vi "禹山溶解氧校准.vi"() -> ()   [LabVIEW 2016, in "斯坦道多参数.lvlib"]
uses:
  <vilib>/Utility/miscctls.llb/LVPointTypeDef.ctl
  <vilib>/Analysis/NI_AALBase.lvlib
  <vilib>/Analysis/NI_AALPro.lvlib
  <vilib>/Utility/config.llb/NI_LVConfig.lvlib
panel:
  out "通讯状态":string
  in  "盐度自动获取":bool
  in  "大气压补偿":dbl format="%#.2f"
  in  "盐度补偿":dbl format="%#.2f"
  out "DO %":dbl caption="饱和度值" format="%#.2f"
  out "第二点校准值":dbl
  out "第一点校准值":dbl
  out "最小值":sgl format="%.2g"
  out "最大值":sgl format="%.2g"
  in  "校准停止":bool
  in  "校准模式":enum16{"两点校准", "单点校准"}(ring)
  in  "标液2":dbl
  in  "标液1":dbl
  out "波形图表":sgl(graph) caption="历史曲线"
  out "温度测量值":dbl caption="温度" format="%#.2f"
  out "变异系数":dbl format="%.6g"
  out "standard deviation":dbl caption="标准差" format="%0.2f"
  out "mean":dbl caption="均值" format="%0.2f"
  out "提示":string
  in  "校准启动":bool
  out "DO mg/L":dbl caption="测试值" format="%#.2f"
  out "电极斜率":dbl format="%#.6f"
  out "电极零点":dbl format="%#.6f"
  # "溶解氧电极设定"
  # "℃"
  # "%"
  # "mg/L"
  # "kPa"
  # "请选择校准模式:"
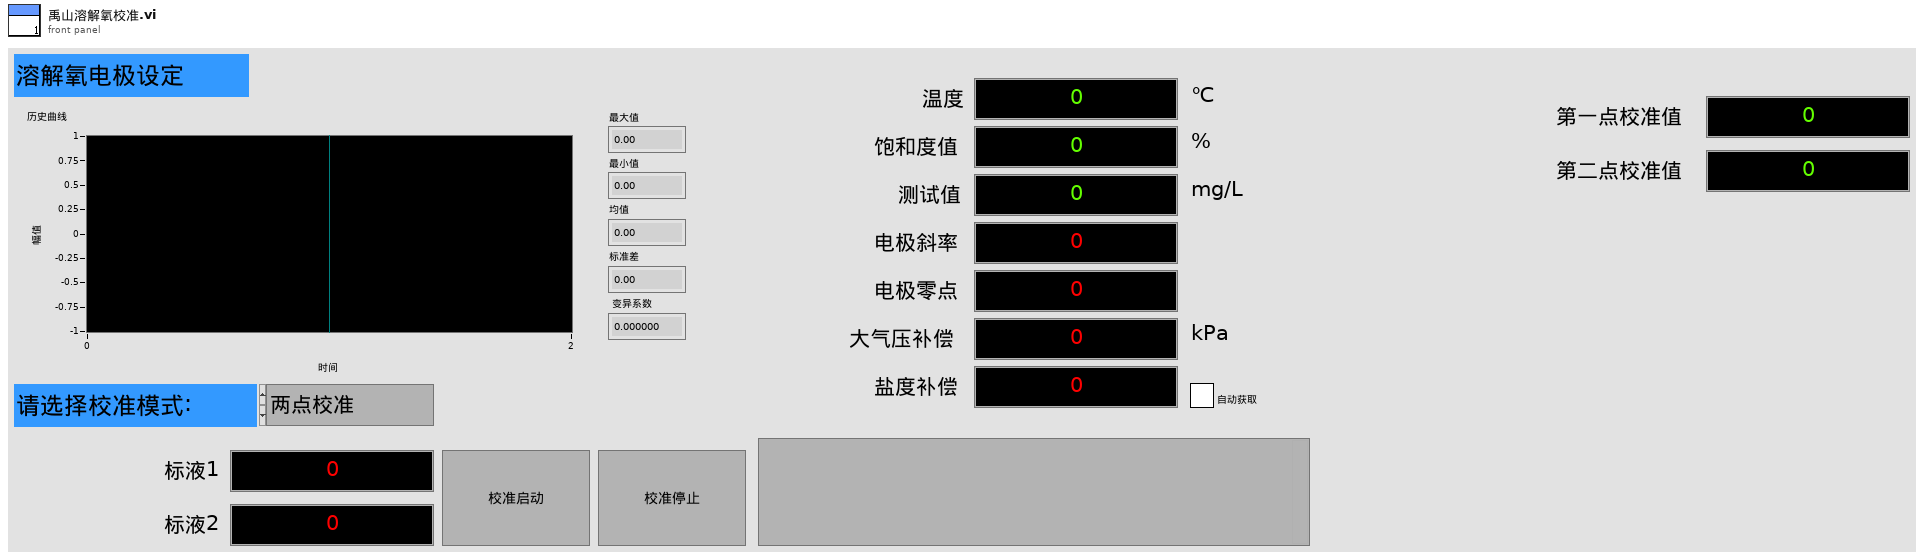
[diagram p1: front panel]
types:
  T1 = typedef "斯坦道多参数.lvlib/校准步骤.ctl" = enum16{"待机", "放置第一点标液", "第一点校准启动", "第一点校准写入", "第一点校准失败", "放置第二点标液", "第二点校准启动", "第二点校准写入", "第二点校准失败", "放置第三点标液", "第三点校准启动", "第三点校准写入", "第三点校准失败", "校准结果写入", "校准结束"}
  T2 = typedef "LVPointTypeDef.ctl" = cluster{"Horizontal":i16, "Vertical":i16}
  T3 = typedef "NI_LVConfig.lvlib/Config Data RefNum.ctl" = refnum<k1>
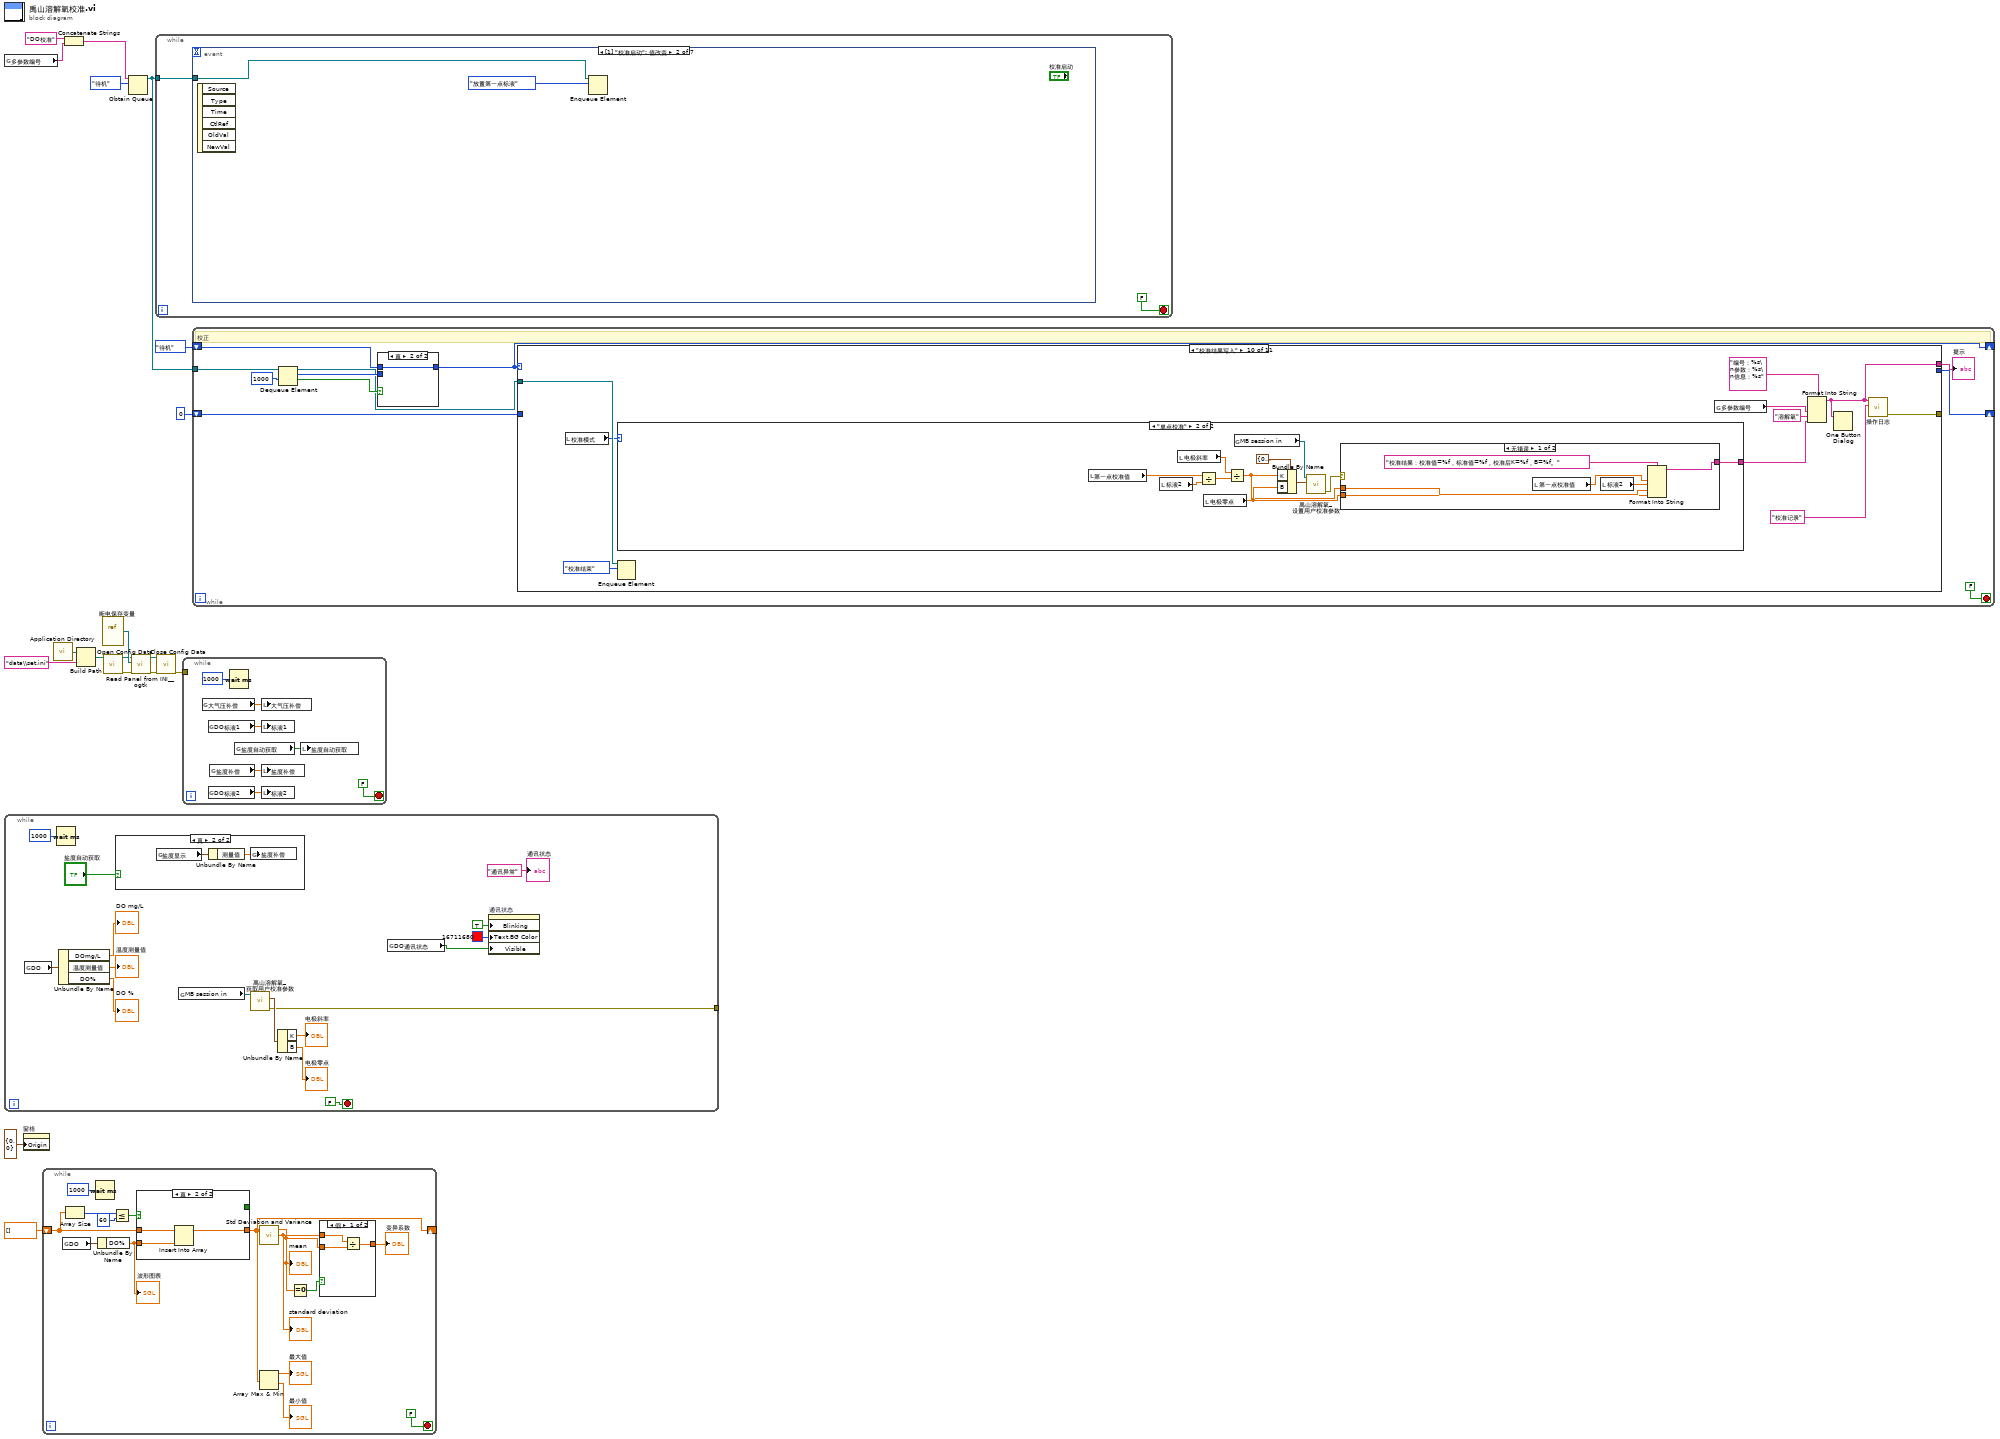
[diagram p0: block diagram]
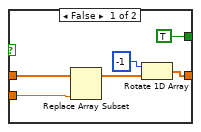
[diagram p3: hidden frame]
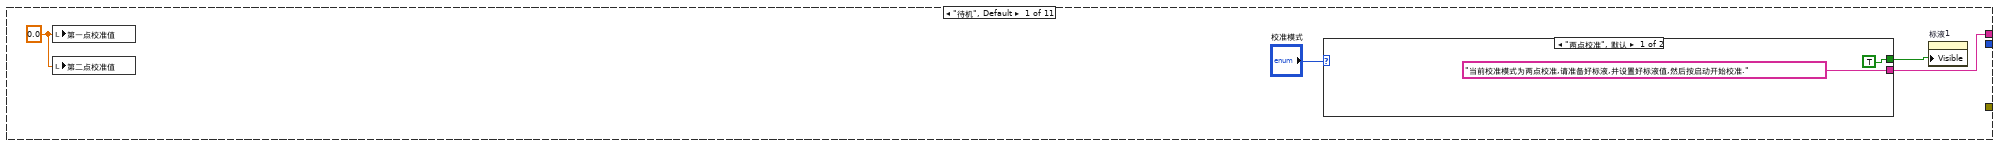
[diagram p5: hidden frame]
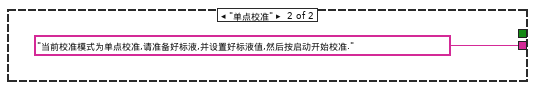
[diagram p6: hidden frame]
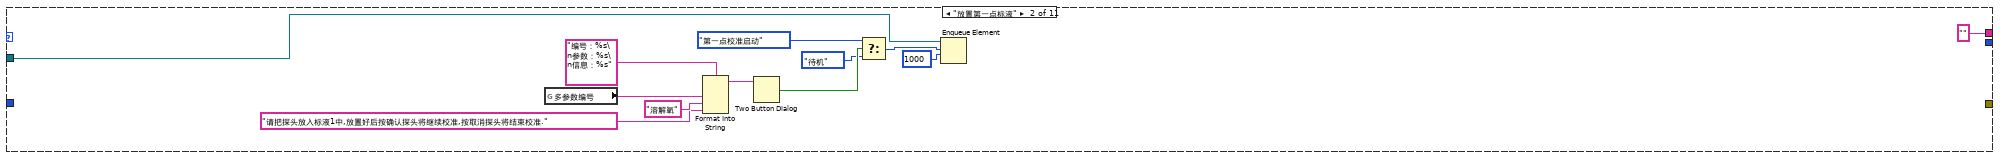
[diagram p7: hidden frame]
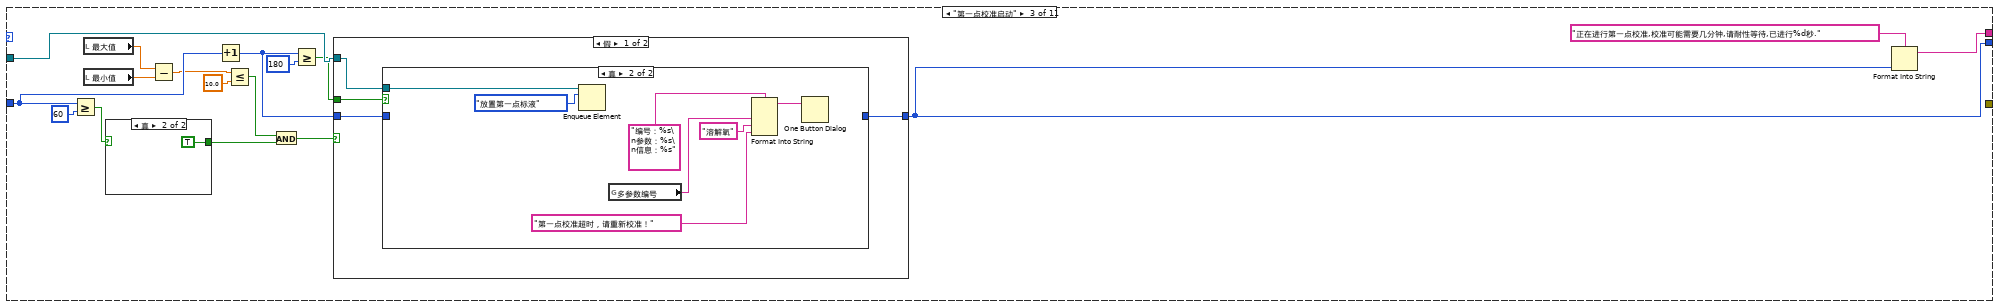
[diagram p8: hidden frame]
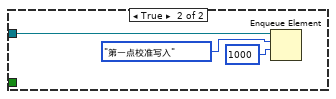
[diagram p10: hidden frame]
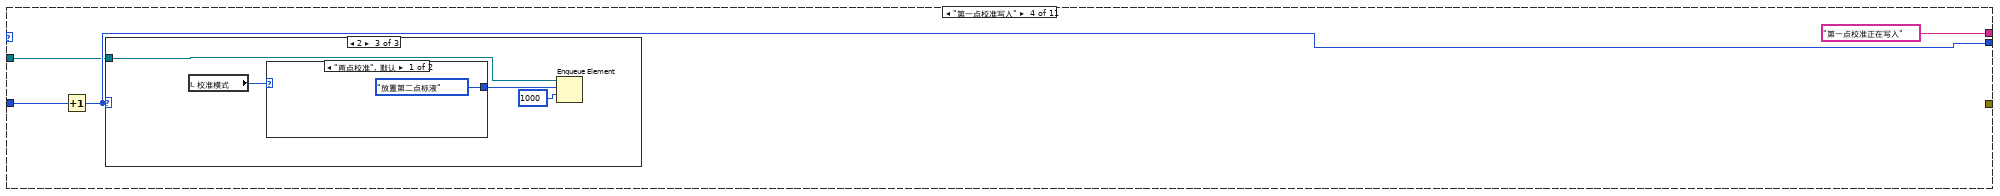
[diagram p12: hidden frame]
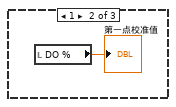
[diagram p14: hidden frame]
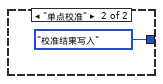
[diagram p15: hidden frame]
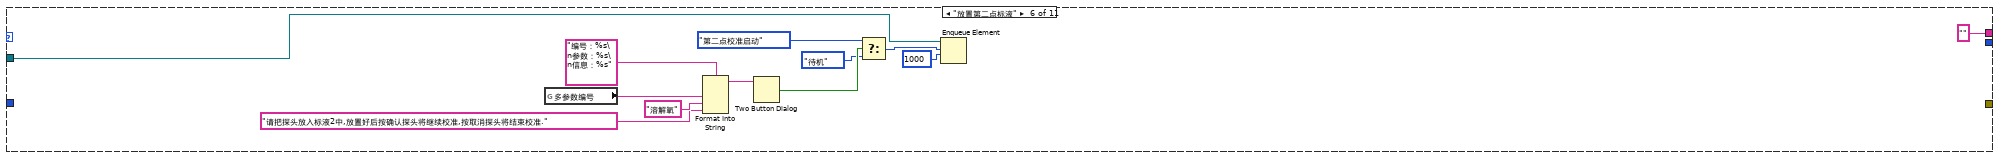
[diagram p17: hidden frame]
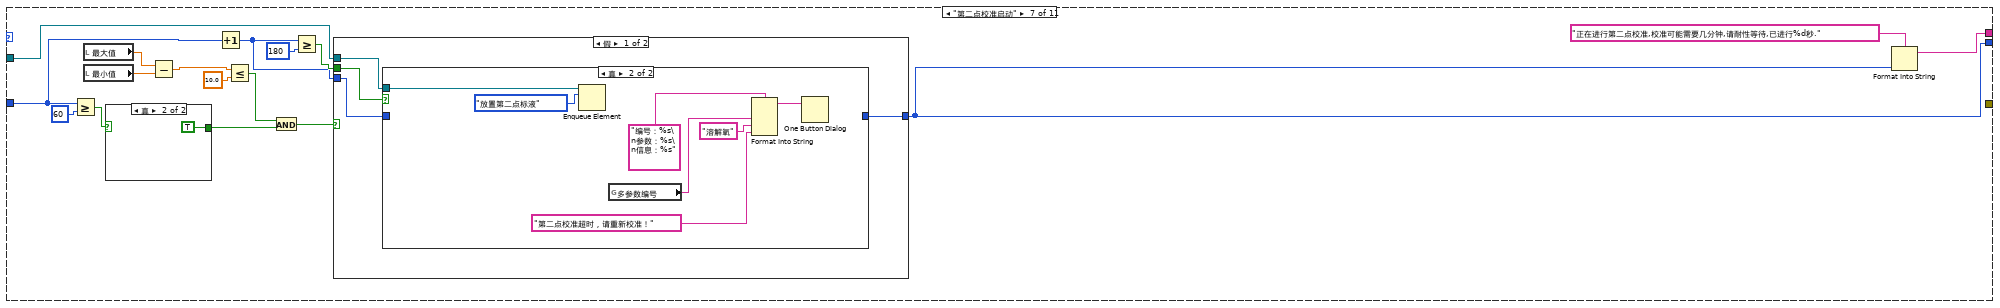
[diagram p18: hidden frame]
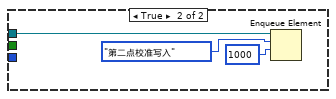
[diagram p20: hidden frame]
diagram:
  n1 = global read "多参数全局变量.vi" "多参数编号"() -> (w1:string)
  n2 = while {
    tunnel: [w29] -> _
    stop <- FALSE stop-if-true
    n3 = global read "禹山过程全局变量.vi" "DO"() -> (w26:cluster{"温度测量值":sgl, "DO%":sgl, "DOmg/L":sgl})
    n4 = Wait (ms)(milliseconds to wait=u32 1000 ("等待时间（毫秒）")) -> ()  [unwired: 1 out]
    n5 = Unbundle By Name(w26) -> ("DOmg/L"=→"DO mg/L":sgl, "温度测量值"=→"温度测量值":sgl, "DO%"=→"DO %":sgl)
    n6 = case shown="真" "盐度自动获取" {
      frame False {
      }
      frame True {
        n7 = global read "多参数全局变量.vi" "盐度显示"() -> (w36:cluster{"温度测量值":sgl, "测量值":sgl, "温度偏移修正值":sgl})
        n8 = Unbundle By Name(w36) -> ("测量值"=w35:sgl)
        n9 = global write "断电保存变量.vi" "盐度补偿"(w35) -> ()
      }
    }
    n10 = global read "多参数全局变量.vi" "MB session in"() -> (w25:refnum<class "MB_Master.lvclass">)
    n11 = call "禹山溶解氧_获取用户校准参数.vi"("MB session in"=w25) -> ("error out"=w29:errorcluster, "输出值"=w32:cluster{"K":sgl, "B":sgl})  [unwired: 8 in, 1 out]
    n12 = Unbundle By Name(w32) -> ("K"=→"电极斜率":sgl, "B"=→"电极零点":sgl)
    n13 = global read "多参数全局变量.vi" "DO通讯状态"() -> (w19:bool)
    n14 = property on="通讯状态" class="Str"("Blinking"=TRUE ("闪烁"), "Text.BG Color"=u32 16711680, "Visible"=w19) -> ()  [unwired: 2 in, 2 out]
    "通讯状态" <- "通讯异常" ("当前串口")
  }
  n15 = property on="窗格" class="Pane"("Origin"=T2 {"Horizontal"=0, "Vertical"=0} ("原点")) -> ()  [unwired: 2 in, 2 out]
  n16 = while {
    shift-right: [w39] -> _
    shift-left: sgl[] [] -> [w47]
    stop <- FALSE stop-if-true
    n17 = global read "禹山过程全局变量.vi" "DO"() -> (w41:cluster{"温度测量值":sgl, "DO%":sgl, "DOmg/L":sgl})
    n18 = Array Size(array=w47) -> (size(s)=w49:i32)
    n19 = Wait (ms)(milliseconds to wait=u32 1000 ("等待时间（毫秒）")) -> ()  [unwired: 1 out]
    n20 = Unbundle By Name(w41) -> ("DO%"=w40:sgl)
    "波形图表" <- w40
    n21 = Less Or Equal?(x=w49, y=60) -> (x <= y?=w48:bool)
    n22 = case shown="真" w48 {
      tunnel: w47 -> [w60 w63]
      tunnel: w40 -> [w58 w62]
      tunnel: [w56 w61] -> w39
      tunnel: [TRUE _] -> _
      frame False {
        n23 = Replace Array Subset(array=w60, new element=w58) -> (w59:sgl[])  [unwired: 1 in]
        n24 = Rotate 1D Array(1:w59, 2:-1 ("n")) -> (0:w56:sgl[])
      }
      frame True {
        n25 = Insert Into Array(array=w63, new element=w62) -> (w61:sgl[])  [unwired: 1 in]
      }
    }
    n26 = call <vilib>:"Std Deviation and Variance.vi"("X"=w39) -> ("mean"=w42:dbl, "standard deviation"=w43:dbl)  [unwired: 1 in, 1 out]
    "standard deviation" <- w43
    "mean" <- w42
    n27 = Array Max & Min(array=w39) -> (max value=→"最大值":sgl, min value=→"最小值":sgl)  [unwired: 2 out]
    n28 = Equal To 0?(x=w42) -> (x = 0?=w46:bool)
    n29 = case shown="假" w46 {
      tunnel: w43 -> [w54 _]
      tunnel: [w53 _] -> w45
      tunnel: w42 -> [w52 _]
      frame False {
        n30 = Divide(x=w54, y=w52) -> (x/y=w53:dbl)
      }
      frame True {
      }
    }
    "变异系数" <- w45
  }
  n31 = call <vilib>:"Application Directory.vi"() -> ("Application Directory"=w9:path)
  n32 = Concatenate Strings("DO校准" ("名称（未命名）"), w1) -> (w2:string)
  n33 = Build Path(base path=w9, name or relative path="data\\set.ini" ("名称或相对路径")) -> (appended path=w10:path)
  n34 = vi-ref "断电保存变量.vi"() -> (w12:refnum<vi>)
  n35 = call <vilib>:"Open Config Data.vi"("configuration file path"=w10) -> ("error out"=w6:errorcluster, "refnum"=w5:T3)  [unwired: 8 in, 1 out]
  n36 = Obtain Queue(name (unnamed)=w2, element data type=校准步骤."待机" ("枚举")) -> (queue out=w13:refnum<queue>)  [unwired: 3 in, 2 out]
  n37 = call <userlib>:"Read Panel from INI__ogtk.vi"("error in (no error)"=w6, "VI ref"=w12, "refnum"=w5) -> ("error out"=w8:errorcluster, "refnum out"=w7:T3)  [unwired: 7 in]
  n38 = while {
    tunnel: w13 -> [w64]
    stop <- FALSE stop-if-true
    n39 = event shown="[1] \"校准启动\": 值改变" {
      selector: _ -> [_ _ _ _ _ _ _]
      dyn-events: _ -> [_ _ _ _ _ _ _]
      timeout: _ -> [_ _ _ _ _ _ _]
      tunnel: w64 -> [_ w67 w71 _ _ _ _]
      event Timeout {
        n40 = event-data() -> ()  [unwired: 1 in, 3 out]
      }
      event "校准启动": Value Change {
        n41 = event-data() -> ()  [unwired: 1 in, 6 out]
        n42 = Enqueue Element(queue=w67, element=校准步骤."放置第一点标液" ("元素")) -> ()  [unwired: 2 in, 3 out]
      }
      event "校准停止": Value Change {
        n43 = event-data() -> ()  [unwired: 1 in, 6 out]
        n44 = Flush Queue(queue=w71) -> (queue out=w68:refnum<queue>)  [unwired: 1 in, 2 out]
        n45 = Enqueue Element(queue=w68, element=校准步骤."待机" ("元素"), timeout in ms (-1)=1000 ("超时毫秒(-1)")) -> ()  [unwired: 1 in, 3 out]
      }
      event "电极零点", "电极斜率", "标液1", "标液2", "大气压补偿": Mouse Down {
        n46 = event-data() -> ("CtlRef"=w72:refnum<vi>)  [unwired: 1 in, 7 out]
        n47 = property class="DigNum (严格)"(reference=w72) -> (reference out=w73:refnum<vi>, "Value"=w74:dbl)  [unwired: 1 in, 1 out]
        n48 = call "数字键盘.vi"("OldNumber"=w74) -> ("NewNumber"=w75:dbl)  [unwired: 1 in]
        n49 = property class="DigNum (严格)"(reference=w73, "Val(Sgnl)"=w75) -> ()  [unwired: 1 in, 2 out]
      }
      event "盐度补偿": Mouse Down {
        n50 = event-data() -> ("CtlRef"=w77:refnum<vi>)  [unwired: 1 in, 7 out]
        n51 = local read "盐度自动获取"() -> (w76:bool)
        n52 = case shown="假" w76 {
          tunnel: w77 -> [w78 _]
          frame False {
            n53 = property class="DigNum (严格)"(reference=w78) -> (reference out=w79:refnum<vi>, "Value"=w80:dbl)  [unwired: 1 in, 1 out]
            n54 = call "数字键盘.vi"("OldNumber"=w80) -> ("NewNumber"=w81:dbl)  [unwired: 1 in]
            n55 = property class="DigNum (严格)"(reference=w79, "Val(Sgnl)"=w81) -> ()  [unwired: 1 in, 2 out]
          }
          frame True {
          }
        }
      }
      event "电极零点", "电极斜率": Value Change {
        n56 = event-data() -> ()  [unwired: 1 in, 6 out]
        n57 = local read "电极斜率"() -> (w84:dbl)
        n58 = local read "电极零点"() -> (w83:dbl)
        n59 = global read "多参数全局变量.vi" "MB session in"() -> (w82:refnum<class "MB_Master.lvclass">)
        n60 = Bundle By Name(cluster=cluster{"K":sgl, "B":sgl} {"K"=0.0, "B"=0.0} ("用户校准参数"), "K"=w84, "B"=w83) -> (w85:cluster{"K":sgl, "B":sgl})
        n61 = call "禹山溶解氧_设置用户校准参数.vi"("用户校准参数"=w85, "MB session in"=w82) -> ()  [unwired: 8 in, 2 out]
      }
      event "标液1", "标液2", "盐度补偿", "大气压补偿", "盐度自动获取": Value Change {
        n62 = event-data() -> ()  [unwired: 1 in, 6 out]
        n63 = flat-sequence {
          frame #0 {
            n64 = local read "盐度自动获取"() -> (w87:bool)
            n65 = global write "断电保存变量.vi" "盐度补偿"("盐度补偿") -> ()
            n66 = global write "断电保存变量.vi" "DO标液1"("标液1") -> ()
            n67 = global write "断电保存变量.vi" "DO标液2"("标液2") -> ()
            n68 = global write "断电保存变量.vi" "大气压补偿"("大气压补偿") -> ()
            n69 = global write "断电保存变量.vi" "盐度自动获取"(w87) -> ()
          }
          frame #1 {
            n70 = call <vilib>:"Application Directory.vi"() -> ("Application Directory"=w101:path)
            n71 = Build Path(base path=w101, name or relative path="data\\set.ini" ("名称或相对路径")) -> (appended path=w100:path)
            n72 = call <vilib>:"Open Config Data.vi"("configuration file path"=w100) -> ("error out"=w104:errorcluster, "refnum"=w105:T3)  [unwired: 8 in, 1 out]
            n73 = vi-ref "断电保存变量.vi"() -> (w98:refnum<vi>)
            n74 = call <userlib>:"Write Panel to INI__ogtk.vi"("error in (no error)"=w104, "VI ref"=w98, "refnum"=w105) -> ("error out"=w102:errorcluster, "refnum out"=w103:T3)  [unwired: 7 in]
            n75 = call <vilib>:"Close Config Data.vi"("error in (no error)"=w102, "refnum"=w103) -> ("error out"=w94:errorcluster, "file path"=w95:path)  [unwired: 8 in]
            n76 = Open/Create/Replace File(file path (use dialog)=w95, error in=w94) -> (refnum out=w96:refnum<file>, error out=w97:errorcluster)  [unwired: 4 in, 1 out]
            n77 = Flush File(refnum=w96, error in=w97) -> (refnum out=w92:refnum<file>, error out=w93:errorcluster)
            n78 = Close File(refnum=w92, error in=w93) -> ()  [unwired: 2 out]
          }
        }
      }
    }
  }
  n79 = call <vilib>:"Close Config Data.vi"("error in (no error)"=w8, "refnum"=w7) -> ("error out"=w4:errorcluster)  [unwired: 8 in, 1 out]
  n80 = while {
    tunnel: w4 -> [_]
    stop <- FALSE stop-if-true
    n81 = global read "断电保存变量.vi" "大气压补偿"() -> (w108:dbl)
    n82 = global read "断电保存变量.vi" "DO标液1"() -> (w110:dbl)
    n83 = global read "断电保存变量.vi" "DO标液2"() -> (w109:dbl)
    n84 = global read "断电保存变量.vi" "盐度补偿"() -> (w106:dbl)
    n85 = Wait (ms)(milliseconds to wait=u32 1000 ("等待时间（毫秒）")) -> ()  [unwired: 1 out]
    n86 = global read "断电保存变量.vi" "盐度自动获取"() -> (w107:bool)
    n87 = local write "大气压补偿"(w108) -> ()
    n88 = local write "标液1"(w110) -> ()
    n89 = local write "盐度补偿"(w106) -> ()
    n90 = local write "标液2"(w109) -> ()
    n91 = local write "盐度自动获取"(w107) -> ()
  }
  n92 = while "While循环" {
    shift-right: [w114] -> _
    shift-left: 校准步骤."待机" ("枚举") -> [w115]
    shift-right: [w121] -> _
    shift-left: 0 -> [w122]
    tunnel: w13 -> [w119]
    stop <- FALSE stop-if-true
    # "校正"
    n93 = Dequeue Element(queue=w119, timeout in ms (-1)=1000 ("超时毫秒(-1)")) -> (queue out=w113:refnum<queue>, element=w116:T1, timed out?=w117:bool)  [unwired: 1 in, 1 out]
    n94 = case shown="真" w117 {
      tunnel: w116 -> [w124 _]
      tunnel: [w124 w125] -> w114
      tunnel: w115 -> [_ w125]
      frame False {
      }
      frame True {
      }
    }
    n95 = case shown="\"校准结果写入\"" w114 {
      tunnel: [w129 "" ("提示") w160 "第一点校准正在写入" ("提示") _ "" ("提示") w216 "第二点校准正在写入" ("提示") _ w244 w301] -> w120
      tunnel: w122 -> [_ _ w154 w180 _ _ w210 w236 _ _ _]
      tunnel: [_ _ w145 w179 _ _ w201 w235 _ _ _] -> w121
      tunnel: w113 -> [_ w144 w148 w178 _ w200 w204 w234 _ w251 _]
      tunnel: [_ _ _ _ _ _ _ _ _ w248 _] -> _
      frame "待机", Default {
        w126 = 0.0 ("第一点校准值")
        n96 = local write "第一点校准值"(w126) -> ()
        n97 = local write "第二点校准值"(w126) -> ()
        n98 = case shown="\"两点校准\", 默认" "校准模式" {
          tunnel: ["当前校准模式为两点校准,请准备好标液,并设置好标液值,然后按启动开始校准." ("提示") "当前校准模式为单点校准,请准备好标液,并设置好标液值,然后按启动开始校准." ("提示")] -> w129
          tunnel: [TRUE ("可见") _] -> w127
          frame "两点校准", Default {
          }
          frame "单点校准" {
          }
        }
        n99 = property on="标液1" class="DigNum (严格)"("Visible"=w127) -> ()  [unwired: 2 in, 2 out]
      }
      frame "放置第一点标液" {
        n100 = global read "多参数全局变量.vi" "多参数编号"() -> (w136:string)
        n101 = Format Into String(format string="编号：%s\n参数：%s\n信息：%s" ("格式字符串"), w136, "溶解氧" ("输入 2"), "请把探头放入标液1中,放置好后按确认探头将继续校准,按取消探头将结束校准." ("消息")) -> (resulting string=w133:string)  [unwired: 2 in, 1 out]
        n102 = Two Button Dialog(message=w133) -> (T button?=w142:bool)  [unwired: 2 in]
        n103 = Select(t=校准步骤."第一点校准启动" ("元素"), s=w142, f=校准步骤."待机" ("元素")) -> (s? t:f=w139:T1)
        n104 = Enqueue Element(queue=w144, element=w139, timeout in ms (-1)=1000 ("超时毫秒(-1)")) -> ()  [unwired: 1 in, 3 out]
      }
      frame "第一点校准启动" {
        n105 = Greater Or Equal?(x=w154, y=60) -> (x >= y?=w155:bool)
        n106 = local read "最大值"() -> (w151:sgl)
        n107 = local read "最小值"() -> (w152:sgl)
        n108 = case shown="真" w155 {
          tunnel: [_ TRUE] -> w153
          frame False {
          }
          frame True {
          }
        }
        n109 = Subtract(x=w151, y=w152) -> (x-y=w150:sgl)
        n110 = Increment(x=w154) -> (x+1=w146:i32)
        n111 = Less Or Equal?(x=w150, y=10.0) -> (x <= y?=w158:bool)
        n112 = And(x=w158, y=w153) -> (x .and. y?=w149:bool)
        n113 = Greater Or Equal?(x=w146, y=180) -> (x >= y?=w147:bool)
        n114 = case shown="假" w149 {
          tunnel: w148 -> [w164 w176]
          tunnel: w147 -> [w165 _]
          tunnel: w146 -> [w163 _]
          tunnel: [w162 _] -> w145
          frame False {
            n115 = case shown="真" w165 {
              tunnel: w164 -> [_ w173]
              tunnel: w163 -> [w166 _]
              tunnel: [w166 _] -> w162
              frame False {
              }
              frame True {
                n116 = Enqueue Element(queue=w173, element=校准步骤."放置第一点标液" ("元素")) -> ()  [unwired: 2 in, 3 out]
                n117 = global read "多参数全局变量.vi" "多参数编号"() -> (w170:string)
                n118 = Format Into String(format string="编号：%s\n参数：%s\n信息：%s" ("格式字符串"), w170, "溶解氧" ("输入 2"), "第一点校准超时，请重新校准！" ("error source (\" \")")) -> (resulting string=w168:string)  [unwired: 2 in, 1 out]
                n119 = One Button Dialog(message=w168) -> ()  [unwired: 1 in, 1 out]
              }
            }
          }
          frame True {
            n120 = Enqueue Element(queue=w176, element=校准步骤."第一点校准写入" ("元素"), timeout in ms (-1)=1000 ("超时毫秒(-1)")) -> ()  [unwired: 1 in, 3 out]
          }
        }
        n121 = Format Into String(format string="正在进行第一点校准,校准可能需要几分钟,请耐性等待,已进行%d秒." ("格式字符串"), w145) -> (resulting string=w160:string)  [unwired: 2 in, 1 out]
      }
      frame "第一点校准写入" {
        n122 = Increment(x=w180) -> (x+1=w179:i32)
        n123 = case shown="2" w179 {
          tunnel: w178 -> [_ _ w186]
          frame 0, Default {
          }
          frame 1 {
            n124 = local read "DO %"() -> (→"第一点校准值":dbl)
          }
          frame 2 {
            n125 = local read "校准模式"() -> (w185:enum16{"两点校准", "单点校准"})
            n126 = case shown="\"两点校准\", 默认" w185 {
              tunnel: [校准步骤."放置第二点标液" ("元素") 校准步骤."校准结果写入" ("元素")] -> w184
              frame "两点校准", Default {
              }
              frame "单点校准" {
              }
            }
            n127 = Enqueue Element(queue=w186, element=w184, timeout in ms (-1)=1000 ("超时毫秒(-1)")) -> ()  [unwired: 1 in, 3 out]
          }
        }
      }
      frame "第一点校准失败" {
      }
      frame "放置第二点标液" {
        n128 = global read "多参数全局变量.vi" "多参数编号"() -> (w192:string)
        n129 = Format Into String(format string="编号：%s\n参数：%s\n信息：%s" ("格式字符串"), w192, "溶解氧" ("输入 2"), "请把探头放入标液2中,放置好后按确认探头将继续校准,按取消探头将结束校准." ("消息")) -> (resulting string=w189:string)  [unwired: 2 in, 1 out]
        n130 = Two Button Dialog(message=w189) -> (T button?=w198:bool)  [unwired: 2 in]
        n131 = Select(t=校准步骤."第二点校准启动" ("元素"), s=w198, f=校准步骤."待机" ("元素")) -> (s? t:f=w195:T1)
        n132 = Enqueue Element(queue=w200, element=w195, timeout in ms (-1)=1000 ("超时毫秒(-1)")) -> ()  [unwired: 1 in, 3 out]
      }
      frame "第二点校准启动" {
        n133 = Greater Or Equal?(x=w210, y=60) -> (x >= y?=w211:bool)
        n134 = local read "最大值"() -> (w207:sgl)
        n135 = local read "最小值"() -> (w208:sgl)
        n136 = case shown="真" w211 {
          tunnel: [_ TRUE] -> w209
          frame False {
          }
          frame True {
          }
        }
        n137 = Subtract(x=w207, y=w208) -> (x-y=w206:sgl)
        n138 = Increment(x=w210) -> (x+1=w202:i32)
        n139 = Less Or Equal?(x=w206, y=10.0) -> (x <= y?=w214:bool)
        n140 = And(x=w214, y=w209) -> (x .and. y?=w205:bool)
        n141 = Greater Or Equal?(x=w202, y=180) -> (x >= y?=w203:bool)
        n142 = case shown="假" w205 {
          tunnel: w204 -> [w220 w232]
          tunnel: w203 -> [w221 _]
          tunnel: w202 -> [w219 _]
          tunnel: [w218 _] -> w201
          frame False {
            n143 = case shown="真" w221 {
              tunnel: w220 -> [_ w229]
              tunnel: w219 -> [w222 _]
              tunnel: [w222 _] -> w218
              frame False {
              }
              frame True {
                n144 = Enqueue Element(queue=w229, element=校准步骤."放置第二点标液" ("元素")) -> ()  [unwired: 2 in, 3 out]
                n145 = global read "多参数全局变量.vi" "多参数编号"() -> (w226:string)
                n146 = Format Into String(format string="编号：%s\n参数：%s\n信息：%s" ("格式字符串"), w226, "溶解氧" ("输入 2"), "第二点校准超时，请重新校准！" ("error source (\" \")")) -> (resulting string=w224:string)  [unwired: 2 in, 1 out]
                n147 = One Button Dialog(message=w224) -> ()  [unwired: 1 in, 1 out]
              }
            }
          }
          frame True {
            n148 = Enqueue Element(queue=w232, element=校准步骤."第二点校准写入" ("元素"), timeout in ms (-1)=1000 ("超时毫秒(-1)")) -> ()  [unwired: 1 in, 3 out]
          }
        }
        n149 = Format Into String(format string="正在进行第二点校准,校准可能需要几分钟,请耐性等待,已进行%d秒." ("格式字符串"), w201) -> (resulting string=w216:string)  [unwired: 2 in, 1 out]
      }
      frame "第二点校准写入" {
        n150 = Increment(x=w236) -> (x+1=w235:i32)
        n151 = case shown="2" w235 {
          tunnel: w234 -> [_ _ w241]
          frame 0, Default {
          }
          frame 1 {
            n152 = local read "DO %"() -> (→"第二点校准值":dbl)
          }
          frame 2 {
            n153 = Enqueue Element(queue=w241, element=校准步骤."校准结果写入" ("元素"), timeout in ms (-1)=1000 ("超时毫秒(-1)")) -> ()  [unwired: 1 in, 3 out]
          }
        }
      }
      frame "第二点校准失败" {
      }
      frame "校准结果写入" {
        n154 = local read "校准模式"() -> (w249:enum16{"两点校准", "单点校准"})
        n155 = case shown="\"单点校准\"" w249 {
          tunnel: [w261 w283] -> w243
          frame "两点校准", Default {
            n156 = local read "第一点校准值"() -> (w272:dbl)
            n157 = local read "第二点校准值"() -> (w271:dbl)
            n158 = local read "标液1"() -> (w269:dbl)
            n159 = local read "标液2"() -> (w268:dbl)
            n160 = Insert Into Array(array=dbl[] [] ("Weight"), new element #1=w269, new element #2=w268) -> (w267:dbl[])  [unwired: 1 in]
            n161 = Insert Into Array(array=dbl[] [] ("Weight"), new element #1=w272, new element #2=w271) -> (w266:dbl[])  [unwired: 1 in]
            n162 = call <vilib>:"Linear Fit.vi"("Y"=w267, "X"=w266) -> ("slope"=w260:dbl, "intercept"=w257:dbl)  [unwired: 9 in, 3 out]
            n163 = local read "电极斜率"() -> (w258:dbl)
            n164 = Divide(x=w257, y=100.0) -> (x/y=w253:dbl)
            n165 = local read "电极零点"() -> (w255:dbl)
            n166 = Multiply(x=w260, y=w258) -> (x*y=w259:dbl)
            n167 = Multiply(x=w258, y=w253) -> (x*y=w256:dbl)
            n168 = Add(x=w256, y=w255) -> (x+y=w254:dbl)
            n169 = global read "多参数全局变量.vi" "MB session in"() -> (w265:refnum<class "MB_Master.lvclass">)
            n170 = Bundle By Name(cluster=cluster{"K":sgl, "B":sgl} {"K"=0.0, "B"=0.0} ("用户校准参数"), "K"=w259, "B"=w254) -> (w264:cluster{"K":sgl, "B":sgl})
            n171 = call "禹山溶解氧_设置用户校准参数.vi"("用户校准参数"=w264, "MB session in"=w265) -> ("error out"=w262:errorcluster)  [unwired: 8 in, 1 out]
            n172 = case shown="无错误" w262 {
              tunnel: w259 -> [w279 _]
              tunnel: w254 -> [w278 _]
              tunnel: [w277 "校准失败"] -> w261
              frame No Error {
                n173 = local read "第一点校准值"() -> (w281:dbl)
                n174 = local read "第二点校准值"() -> (w275:dbl)
                n175 = local read "标液1"() -> (w276:dbl)
                n176 = local read "标液2"() -> (w274:dbl)
                n177 = Format Into String(format string="校准结果：第一点校准值=%f，第一点标准值=%f；第二点校准值=%f，第二点标准值=%f；校准后K=%f；B=%f。" ("提示"), w281, w276, w275, w274, w279, w278) -> (resulting string=w277:string)  [unwired: 2 in, 1 out]
              }
              frame Error {
              }
            }
          }
          frame "单点校准" {
            n178 = local read "第一点校准值"() -> (w288:dbl)
            n179 = local read "标液2"() -> (w287:dbl)
            n180 = local read "电极斜率"() -> (w285:dbl)
            n181 = Divide(x=w288, y=w287) -> (x/y=w284:dbl)
            n182 = local read "电极零点"() -> (w289:dbl)
            n183 = Divide(x=w285, y=w284) -> (x/y=w286:dbl)
            n184 = global read "多参数全局变量.vi" "MB session in"() -> (w293:refnum<class "MB_Master.lvclass">)
            n185 = Bundle By Name(cluster=cluster{"K":sgl, "B":sgl} {"K"=0.0, "B"=0.0} ("用户校准参数"), "K"=w286, "B"=w289) -> (w292:cluster{"K":sgl, "B":sgl})
            n186 = call "禹山溶解氧_设置用户校准参数.vi"("用户校准参数"=w292, "MB session in"=w293) -> ("error out"=w290:errorcluster)  [unwired: 8 in, 1 out]
            n187 = case shown="无错误" w290 {
              tunnel: w286 -> [w295 _]
              tunnel: w289 -> [w294 _]
              tunnel: [w298 "校准失败"] -> w283
              frame No Error {
                n188 = local read "第一点校准值"() -> (w299:dbl)
                n189 = local read "标液2"() -> (w296:dbl)
                n190 = Format Into String(format string="校准结果：校准值=%f，标准值=%f，校准后K=%f，B=%f。" ("提示"), w299, w296, w295, w294) -> (resulting string=w298:string)  [unwired: 2 in, 1 out]
              }
              frame Error {
              }
            }
          }
        }
        n191 = Enqueue Element(queue=w251, element=校准步骤."校准结束" ("元素")) -> ()  [unwired: 2 in, 3 out]
        n192 = global read "多参数全局变量.vi" "多参数编号"() -> (w246:string)
        n193 = Format Into String(format string="编号：%s\n参数：%s\n信息：%s" ("格式字符串"), w246, "溶解氧" ("输入 2"), w243) -> (resulting string=w244:string)  [unwired: 2 in, 1 out]
        n194 = One Button Dialog(message=w244) -> ()  [unwired: 1 in, 1 out]
        n195 = call "操作日志.vi"("table"="校准记录", "日志信息"=w244) -> ("error out"=w248:errorcluster)  [unwired: 9 in]
      }
      frame "校准结束" {
        n196 = local read "提示"() -> (w301:string)
      }
    }
    "提示" <- w120
  }
